vi "53230AGetHisto.vi"(1 "Channel2":T1={"AutoLevel"=FALSE, "Thresold"=1.0, "Impedance "=1000000.0, "Voltage Range"=5.0, "Active Edge "=1} {"Active Edge" items=["Positive", "Negative"]; "Impedance" items=["50"=50.0, "1E+6"=1000000.0]}, 2 "Channel1":T1={"AutoLevel"=FALSE, "Thresold"=1.0, "Impedance "=1000000.0, "Voltage Range"=5.0, "Active Edge "=1} {"Active Edge" items=["Positive", "Negative"]; "Impedance" items=["50"=50.0, "1E+6"=1000000.0]}, 3 "Numeric Control":i32) -> (0 "Measurements":dbl[](array[numeric]) format="%#_12g")   [LabVIEW 2014]
uses:
  Configs/Count/Channel.ctl
  <instrlib>/Agilent 532XX Series/Public/Configure/Measurement/Configure Measurement (Time Interval).vi
  <instrlib>/Agilent 532XX Series/Public/Configure/Configure Channel (Auto Threshold Voltage).vi
  <instrlib>/Agilent 532XX Series/Public/Configure/Configure Channel (Slop).vi
  <instrlib>/Agilent 532XX Series/Public/Configure/Configure Channel (Basic).vi
  <instrlib>/Agilent 532XX Series/Public/Configure/Configure Channel (Voltage Range).vi
  <instrlib>/Agilent 532XX Series/Public/Configure/Configure Channel (Threshold Voltage).vi
  <instrlib>/Agilent 532XX Series/Public/Data/Read Measurement (Multiple).vi
  <instrlib>/Agilent 532XX Series/Agilent 532XX Series.lvlib
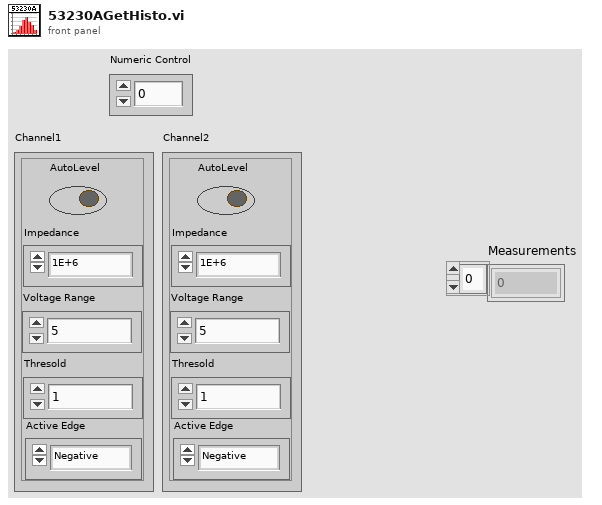
[diagram p1: front panel]
types:
  T1 = typedef "Channel.ctl" = cluster{"AutoLevel":bool, "Thresold":dbl, "Impedance ":dbl, "Voltage Range":dbl, "Active Edge ":i32}
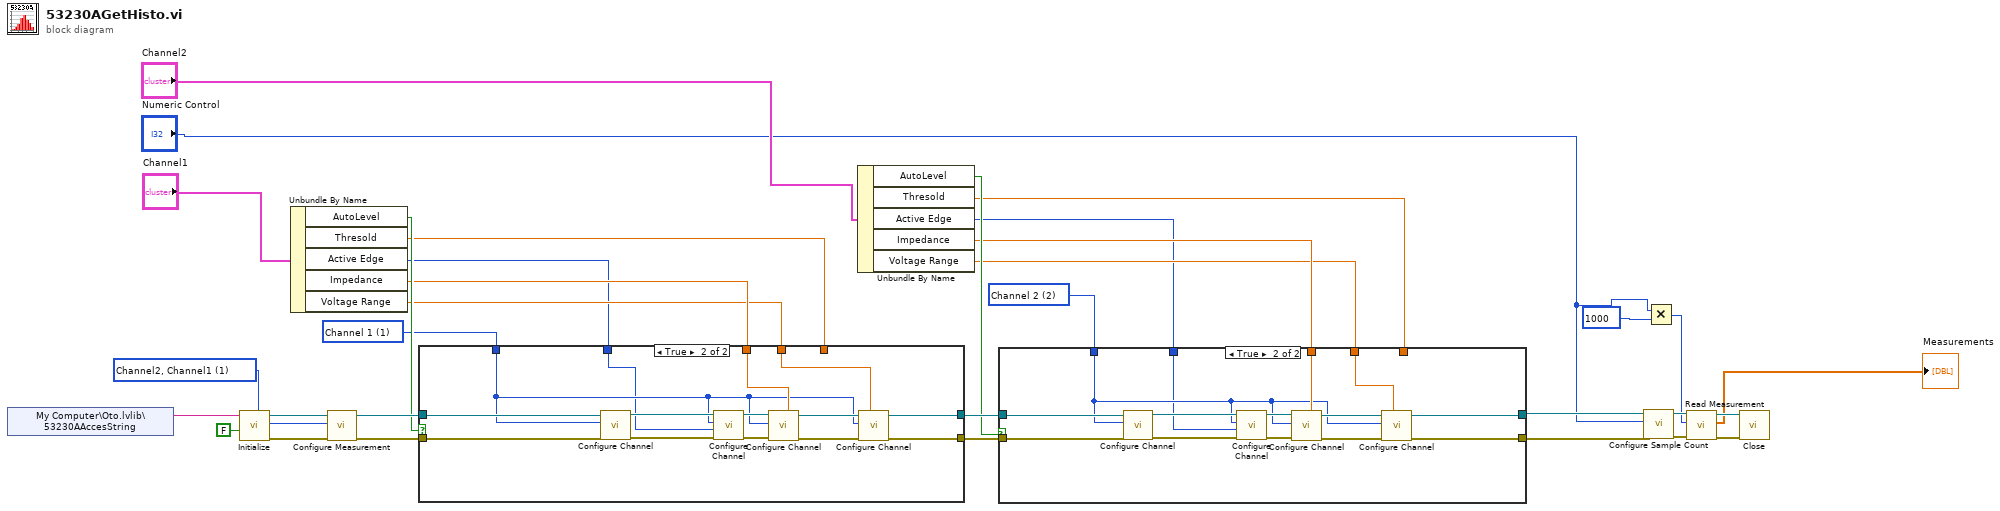
[diagram p0: block diagram]
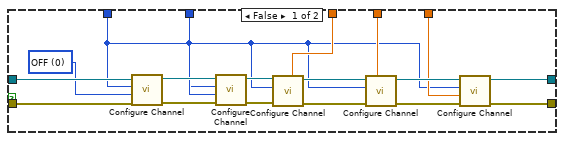
[diagram p2: hidden frame]
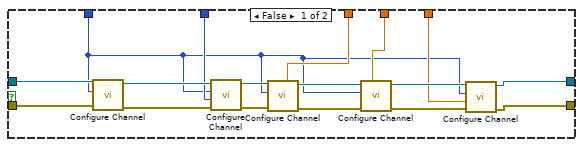
[diagram p3: hidden frame]
diagram:
  w4 = 1 items=["Channel1, Channel2", "Channel2, Channel1", " Channel1", "Channel2"] ("Measurement Channels (0: Channel1, Channel2)")
  w17 = 2 items=["Channel 1"=1, "Channel 2"=2] ("Channel (1: Channel 1)")
  w21 = 1 items=["Channel 1"=1, "Channel 2"=2] ("Channel (1: Channel 1)")
  n1 = shared-variable "My Computer\\Oto.lvlib\\53230AAccesString"() -> (w5:string)  [unwired: 1 in, 1 out]
  n2 = call <instrlib>:"Initialize.vi"("Reset (True)"=FALSE, "VISA resource name"=w5) -> ("error out"=w32:errorcluster, "VISA resource name out"=w31:refnum<visa-resource-name>)  [unwired: 8 in]
  n3 = Unbundle By Name("Channel1") -> ("AutoLevel"=w24:bool, "Thresold"=w14:dbl, "Active Edge"=w16:i32, "Impedance"=w23:dbl, "Voltage Range"=w22:dbl)
  n4 = call-poly <instrlib>:"Configure Measurement.vi"("error in (no error)"=w32, "Measurement Channels (0: Channel1, Channel2)"=w4, "VISA resource name"=w31) -> ("error out"=w27:errorcluster, "VISA resource name out"=w28:refnum<visa-resource-name>)  [unwired: 7 in]
  n5 = case shown="True" w24 {
    tunnel: w28 -> [w44 w64]
    tunnel: w27 -> [w43 w60]
    tunnel: [w40 w56] -> w26
    tunnel: [w39 w55] -> w25
    tunnel: w23 -> [w36 w54]
    tunnel: w22 -> [w37 w53]
    tunnel: w21 -> [w34 w52]
    tunnel: w16 -> [w35 w51]
    tunnel: w14 -> [w38 _]
    frame False {
      n6 = call-poly <instrlib>:"Configure Channel.vi"("error in (no error)"=w43, "Channel (1: Channel 1)"=w34, "VISA resource name"=w44) -> ("error out"=w47:errorcluster, "VISA resource name out"=w50:refnum<visa-resource-name>)  [unwired: 7 in]
      n7 = call-poly <instrlib>:"Configure Channel.vi"("error in (no error)"=w47, "Active Edge (1: Negative)"=w35, "Channel (1: Channel 1)"=w34, "VISA resource name"=w50) -> ("error out"=w46:errorcluster, "VISA resource name out"=w49:refnum<visa-resource-name>)  [unwired: 6 in]
      n8 = call-poly <instrlib>:"Configure Channel.vi"("Impedance (1E+6 Ohm)"=w36, "error in (no error)"=w46, "Channel (1: Channel 1)"=w34, "VISA resource name"=w49) -> ("error out"=w45:errorcluster, "VISA resource name out"=w48:refnum<visa-resource-name>)  [unwired: 6 in]
      n9 = call-poly <instrlib>:"Configure Channel.vi"("Voltage Range (5V)"=w37, "error in (no error)"=w45, "Channel (1: Channel 1)"=w34, "VISA resource name"=w48) -> ("error out"=w41:errorcluster, "VISA resource name out"=w42:refnum<visa-resource-name>)  [unwired: 6 in]
      n10 = call-poly <instrlib>:"Configure Channel.vi"("error in (no error)"=w41, "Threshold Voltage (0 V)"=w38, "Channel (1: Channel 1)"=w34, "VISA resource name"=w42) -> ("error out"=w39:errorcluster, "VISA resource name out"=w40:refnum<visa-resource-name>)  [unwired: 6 in]
    }
    frame True {
      n11 = call-poly <instrlib>:"Configure Channel.vi"("error in (no error)"=w60, "Channel (1: Channel 1)"=w52, "VISA resource name"=w64) -> ("error out"=w59:errorcluster, "VISA resource name out"=w63:refnum<visa-resource-name>)  [unwired: 7 in]
      n12 = call-poly <instrlib>:"Configure Channel.vi"("error in (no error)"=w59, "Active Edge (1: Negative)"=w51, "Channel (1: Channel 1)"=w52, "VISA resource name"=w63) -> ("error out"=w58:errorcluster, "VISA resource name out"=w62:refnum<visa-resource-name>)  [unwired: 6 in]
      n13 = call-poly <instrlib>:"Configure Channel.vi"("Impedance (1E+6 Ohm)"=w54, "error in (no error)"=w58, "Channel (1: Channel 1)"=w52, "VISA resource name"=w62) -> ("error out"=w57:errorcluster, "VISA resource name out"=w61:refnum<visa-resource-name>)  [unwired: 6 in]
      n14 = call-poly <instrlib>:"Configure Channel.vi"("Voltage Range (5V)"=w53, "error in (no error)"=w57, "Channel (1: Channel 1)"=w52, "VISA resource name"=w61) -> ("error out"=w55:errorcluster, "VISA resource name out"=w56:refnum<visa-resource-name>)  [unwired: 6 in]
    }
  }
  n15 = Unbundle By Name("Channel2") -> ("AutoLevel"=w20:bool, "Thresold"=w7:dbl, "Active Edge"=w15:i32, "Impedance"=w19:dbl, "Voltage Range"=w18:dbl)
  n16 = case shown="True" w20 {
    tunnel: w26 -> [w76 w90]
    tunnel: w25 -> [w75 w89]
    tunnel: w19 -> [w73 w88]
    tunnel: w18 -> [w72 w87]
    tunnel: w17 -> [w65 w86]
    tunnel: w15 -> [w74 w85]
    tunnel: [w70 w84] -> w11
    tunnel: [w69 w83] -> w10
    tunnel: w7 -> [w66 _]
    frame False {
      w71 = 0 items=["OFF", "ON", "ONCE"] ("Enable Auto-leveling (1: ON)")
      n17 = call-poly <instrlib>:"Configure Channel.vi"("error in (no error)"=w75, "Enable Auto-leveling (1: ON)"=w71, "Channel (1: Channel 1)"=w65, "VISA resource name"=w76) -> ("error out"=w80:errorcluster, "VISA resource name out"=w77:refnum<visa-resource-name>)  [unwired: 6 in]
      n18 = call-poly <instrlib>:"Configure Channel.vi"("error in (no error)"=w80, "Active Edge (1: Negative)"=w74, "Channel (1: Channel 1)"=w65, "VISA resource name"=w77) -> ("error out"=w81:errorcluster, "VISA resource name out"=w78:refnum<visa-resource-name>)  [unwired: 6 in]
      n19 = call-poly <instrlib>:"Configure Channel.vi"("Impedance (1E+6 Ohm)"=w73, "error in (no error)"=w81, "Channel (1: Channel 1)"=w65, "VISA resource name"=w78) -> ("error out"=w82:errorcluster, "VISA resource name out"=w79:refnum<visa-resource-name>)  [unwired: 6 in]
      n20 = call-poly <instrlib>:"Configure Channel.vi"("Voltage Range (5V)"=w72, "error in (no error)"=w82, "Channel (1: Channel 1)"=w65, "VISA resource name"=w79) -> ("error out"=w67:errorcluster, "VISA resource name out"=w68:refnum<visa-resource-name>)  [unwired: 6 in]
      n21 = call-poly <instrlib>:"Configure Channel.vi"("error in (no error)"=w67, "Threshold Voltage (0 V)"=w66, "Channel (1: Channel 1)"=w65, "VISA resource name"=w68) -> ("error out"=w69:errorcluster, "VISA resource name out"=w70:refnum<visa-resource-name>)  [unwired: 6 in]
    }
    frame True {
      n22 = call-poly <instrlib>:"Configure Channel.vi"("error in (no error)"=w89, "Channel (1: Channel 1)"=w86, "VISA resource name"=w90) -> ("error out"=w93:errorcluster, "VISA resource name out"=w96:refnum<visa-resource-name>)  [unwired: 7 in]
      n23 = call-poly <instrlib>:"Configure Channel.vi"("error in (no error)"=w93, "Active Edge (1: Negative)"=w85, "Channel (1: Channel 1)"=w86, "VISA resource name"=w96) -> ("error out"=w92:errorcluster, "VISA resource name out"=w95:refnum<visa-resource-name>)  [unwired: 6 in]
      n24 = call-poly <instrlib>:"Configure Channel.vi"("Impedance (1E+6 Ohm)"=w88, "error in (no error)"=w92, "Channel (1: Channel 1)"=w86, "VISA resource name"=w95) -> ("error out"=w91:errorcluster, "VISA resource name out"=w94:refnum<visa-resource-name>)  [unwired: 6 in]
      n25 = call-poly <instrlib>:"Configure Channel.vi"("Voltage Range (5V)"=w87, "error in (no error)"=w91, "Channel (1: Channel 1)"=w86, "VISA resource name"=w94) -> ("error out"=w83:errorcluster, "VISA resource name out"=w84:refnum<visa-resource-name>)  [unwired: 6 in]
    }
  }
  n26 = call <instrlib>:"Configure Sample Count.vi"("error in (no error)"=w10, "Sample Count (1)"="Numeric Control", "VISA resource name"=w11) -> ("error out"=w8:errorcluster, "VISA resource name out"=w9:refnum<visa-resource-name>)  [unwired: 7 in]
  n27 = Multiply(x="Numeric Control", y=1000) -> (x*y=w2:i32)
  n28 = call-poly <instrlib>:"Read Measurement.vi"("error in (no error)"=w8, "Timeout (10000 ms)"=w2, "VISA resource name"=w9) -> ("error out"=w30:errorcluster, "Measurements"=→"Measurements":dbl[], "VISA resource name out"=w29:refnum<visa-resource-name>)  [unwired: 6 in]
  n29 = call <instrlib>:"Close.vi"("error in (no error)"=w30, "VISA resource name"=w29) -> ()  [unwired: 9 in, 1 out]
